vi "Default App INI.vi"() -> (2 "Default App INI":path)   [LabVIEW 2020, in "Volatus.lvlib"]
uses:
  Volatus.lvlib
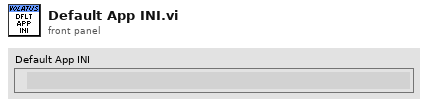
[diagram p1: front panel]
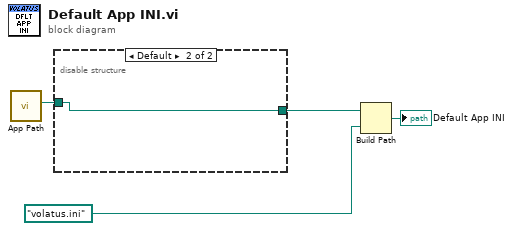
[diagram p0: block diagram]
diagram:
  n1 = call "App Path.vi"() -> ("App Path"=w4:path)  [unwired: 11 in]
  n2 = disable-structure shown="Default" {
    disable-tunnel: w4 -> [w5 w6]
    disable-tunnel: [w5 w6] -> w1
    frame condition #0 {
    }
    frame condition #1 (active) {
    }
  }
  n3 = Build Path(base path=w1, name or relative path=path "volatus.ini") -> (appended path=→"Default App INI":path)
